vi "Write motor by index.vi"(8 "error in (no error)":errorcluster, 9 "index":i32, 10 "Motor.lvclass":refnum<class "Motor.lvclass">, 11 "ICS in":refnum<class "ICS.lvclass">) -> (0 "error out":errorcluster, 3 "ICS out":refnum<class "ICS.lvclass">)   [LabVIEW 2018, in "ICS.lvclass"]
uses:
  ICS.lvclass
  Motor/Motor.lvclass
  ICS.lvclass/ICS.ctl
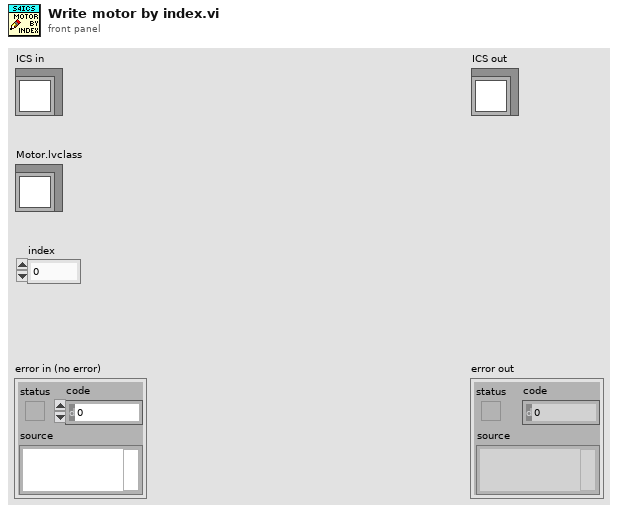
[diagram p1: front panel]
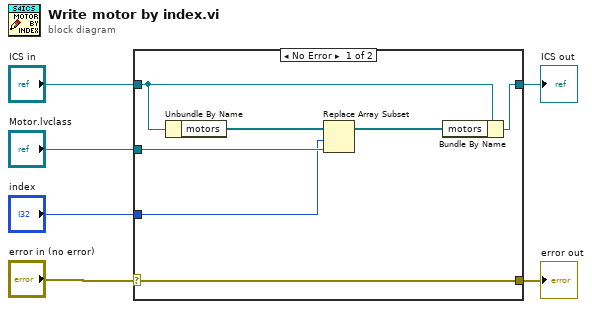
[diagram p0: block diagram]
diagram:
  n1 = case shown="No Error" "error in (no error)" {
    selector: "error in (no error)" -> [w13 w14]
    tunnel: [w13 w14] -> w5
    tunnel: [w12 w15] -> w3
    tunnel: "ICS in" -> [w11 w15]
    tunnel: "Motor.lvclass" -> [w8 _]
    tunnel: "index" -> [w7 _]
    frame No Error {
      n2 = Unbundle By Name(w11) -> ("motors"=w10:refnum<class "Motor.lvclass">[])
      n3 = Replace Array Subset(array=w10, new element=w8, index=w7) -> (w9:refnum<class "Motor.lvclass">[])
      n4 = Bundle By Name(cluster=w11, "motors"=w9) -> (w12:refnum<class "ICS.lvclass">)
    }
    frame Error {
    }
  }
  "error out" <- w5
  "ICS out" <- w3
